vi "SVL Get dB Reference.vi"   [LabVIEW 2017]
doc: "Returns the dB reference stored in the waveform attributes of the scaled signal input. The dB reference is set by the DAQ Assistant for Sound Pressure and Acceleration tasks, the SVL Scale Voltage to EU VI, and the SVL Set dB Reference VI. The dB reference is used for all downstream conversions to dB. Wire data to the <B>scaled signal [EU]</B> input to determine the polymorphic instance to use or manually select the instance."
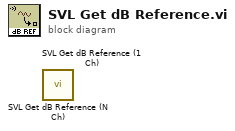
[diagram p0: block diagram]
diagram:
  n1 = call <vilib>:"SVL Get dB Reference (N Ch).vi"() -> ()  [unwired: 9 in, 3 out]
  n2 = call <vilib>:"SVL Get dB Reference (1 Ch).vi"() -> ()  [unwired: 9 in, 3 out]
